vi "Call Read Cal Response.vi"(0 "Port":refnum<visa-resource-name>, 1 "error in":errorcluster) -> (2 "VISA resource name out":refnum<visa-resource-name>, 3 "CAL Complete":bool, 4 "Cal Data":T1={"Time"="18:13:06", "Consecutive good readings"=1, "Total good readings"=3, "A/D counts Sensor 1"=3319.31, "A/D counts Sensor 2"=3319.257, "Diff current/previous Sensor 1"=-0.086, "Diff current/previous Sensor 2"=-0.029}, 5 "error out":errorcluster)   [LabVIEW 2012]
panel:
  in  "Wait":u32=300
  # "Wait 35 seconds to read each CAL response"
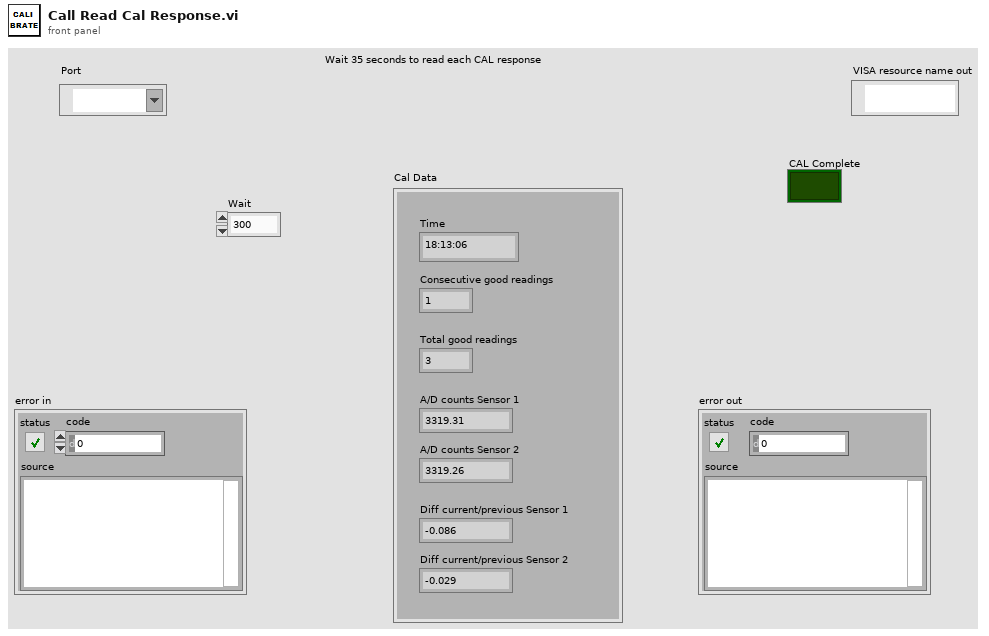
[diagram p1: front panel]
types:
  T1 = cluster{"Time":string, "Consecutive good readings":i32, "Total good readings":i32, "A/D counts Sensor 1":sgl, "A/D counts Sensor 2":sgl, "Diff current/previous Sensor 1":sgl, "Diff current/previous Sensor 2":sgl}
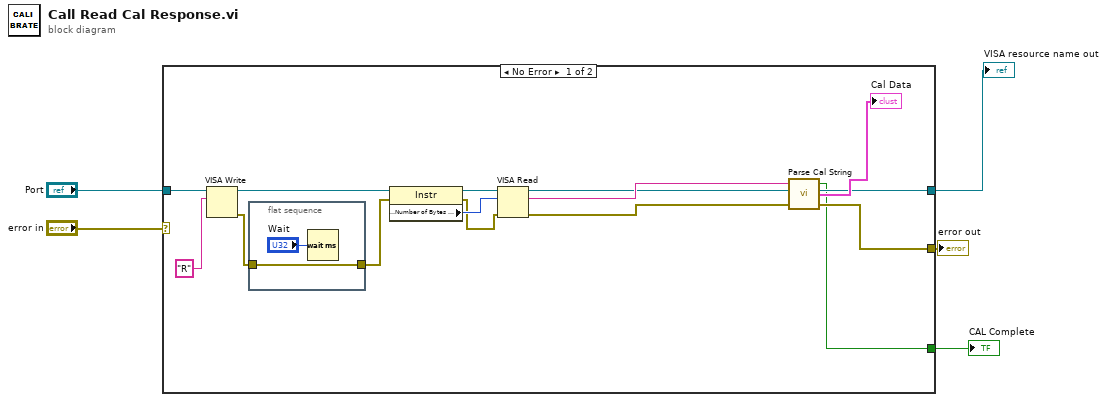
[diagram p0: block diagram]
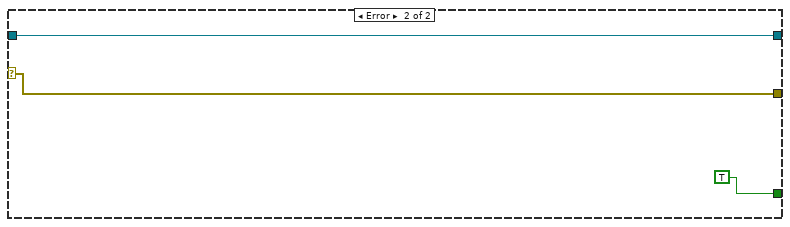
[diagram p2: hidden frame]
diagram:
  n1 = case shown="No Error" "error in" {
    selector: "error in" -> [_ w23]
    tunnel: [w13 w23] -> w5
    tunnel: [w9 w24] -> w4
    tunnel: "Port" -> [w8 w24]
    tunnel: [w7 TRUE] -> w1
    frame No Error {
      n2 = VISA Write(VISA resource name=w8, write buffer="R" ("string")) -> (VISA resource name out=w16:refnum<visa-resource-name>, error out=w15:errorcluster)  [unwired: 1 in, 1 out]
      n3 = flat-sequence {
        tunnel: [w20] -> w14
        tunnel: w15 -> [w20]
        frame #0 {
          n4 = Wait (ms)(milliseconds to wait="Wait") -> ()  [unwired: 1 out]
        }
      }
      n5 = property class="Instr"(reference=w16, error in=w14) -> (reference out=w18:refnum<visa-resource-name>, error out=w17:errorcluster, "Serial Settings:Number of Bytes at Serial Port"=w19:u32)
      n6 = VISA Read(VISA resource name=w18, byte count=w19, error in (no error)=w17) -> (VISA resource name out=w9:refnum<visa-resource-name>, read buffer=w12:string, error out=w10:errorcluster)  [unwired: 1 out]
      n7 = call "Parse Cal String.vi"("error in (no error)"=w10, "read buffer in"=w12) -> ("error out"=w13:errorcluster, "Cal Data"=→"Cal Data":T1, "CAL Complete"=w7:bool)  [unwired: 1 in]
    }
    frame Error {
    }
  }
  "error out" <- w5
  "VISA resource name out" <- w4
  "CAL Complete" <- w1
